vi "getProtocolLevel.vi"(11 "MQTTVersion in":refnum<class "MQTTVersion.lvclass">) -> (2 "Protocol Level":u8 format="%08b", 3 "MQTTVersion out":refnum<class "MQTTVersion.lvclass">)   [LabVIEW 2013, in "MQTT_Control_Packets.lvlib" / "MQTTVersion.lvclass"]
uses:
  MQTTVersion.lvclass
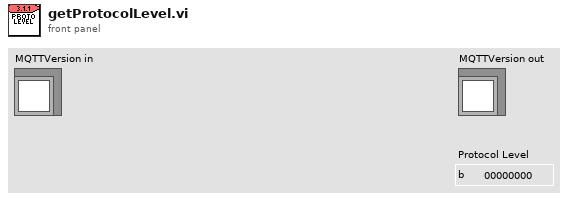
[diagram p1: front panel]
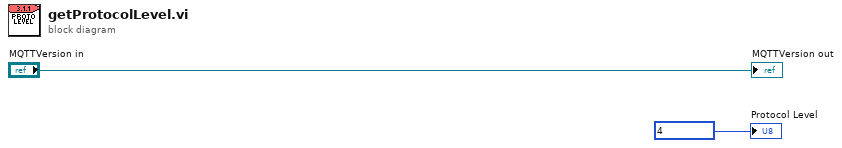
[diagram p0: block diagram]
diagram:
  "MQTTVersion out" <- "MQTTVersion in"
  "Protocol Level" <- u8 4 ("Byte")
